vi "SoftwareBinToFinalData160721.vi"   [LabVIEW 2012]
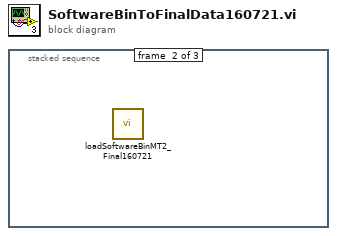
[diagram p0: block diagram]
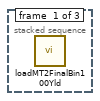
[diagram p2: hidden frame]
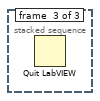
[diagram p3: hidden frame]
diagram:
  n1 = stacked-sequence {
    frame #0 {
      n2 = call "loadMT2FinalBin100Yld.vi"() -> ()  [unwired: 12 in]
    }
    frame #1 {
      n3 = call "loadSoftwareBinMT2_Final160721.vi"() -> ()  [unwired: 12 in]
    }
    frame #2 {
      n4 = Quit LabVIEW() -> ()  [unwired: 1 in]
    }
  }
